vi "FIle_Reader_cl_plot.vi"() -> ()   [LabVIEW 2022 SP3]
panel:
  out "XY Graph 2":cluster{"time 2":dbl[], "Ch0":dbl[]}[](graph)
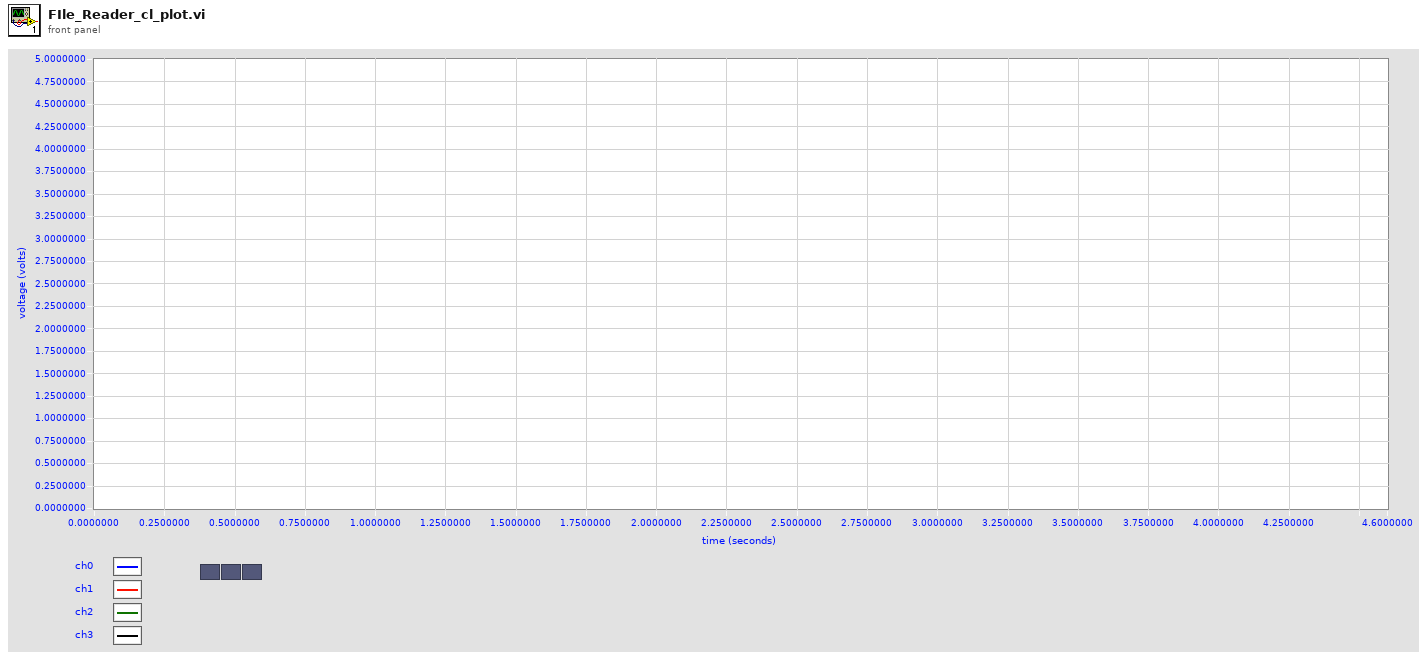
[diagram p1: front panel]
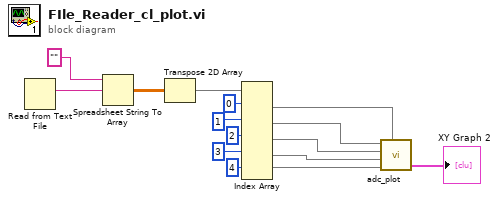
[diagram p0: block diagram]
diagram:
  n1 = Read from Text File() -> (text=w15:string)  [unwired: 4 in, 3 out]
  n2 = Spreadsheet String To Array(format string="", spreadsheet string=w15) -> (array=w1:dbl[][])  [unwired: 2 in]
  n3 = Transpose 2D Array(2D array=w1) -> (transposed array=w8:dbl[][])
  n4 = Index Array "Index Array"(array=w8, index (row) #1=0 ("index"), index (row) #2=1 ("index (row)"), index (row) #3=2 ("index (row)"), index (row) #4=3 ("index (row)"), index (row) #5=4 ("index (row)")) -> (element #1=w11:dbl[], element #2=w10:dbl[], element #3=w5:dbl[], element #4=w4:dbl[], element #5=w2:dbl[])  [unwired: 5 in]
  n5 = call "adc_plot.vi"("Ch0"=w10, "CH1"=w5, "CH2"=w4, "CH3"=w2, "time"=w11) -> ("XY Graph"=→"XY Graph 2":cluster{"time 2":dbl[], "Ch0":dbl[]}[])  [unwired: 2 in]
